vi "Point Data Updated.vi"(8 "error in":errorcluster, 9 "Data":variant, 10 "Point Ident":string, 11 "Sample Photosensor PID Flowsensor PID in":refnum<class "Sample Photosensor PID Flowsensor PID.lvclass">) -> (0 "error out":errorcluster, 3 "Sample Photosensor PID Flowsensor PID out":refnum<class "Sample Photosensor PID Flowsensor PID.lvclass">)   [LabVIEW 2023, in "Sample Photosensor PID Flowsensor PID.lvlib" / "Sample Photosensor PID Flowsensor PID.lvclass"]
uses:
  Sample Photosensor PID Flowsensor PID.lvclass
  Sample Photosensor PID Flowsensor PID.lvclass/Sample Photosensor PID Flowsensor PID.ctl
  <vilib>/Utility/error.llb/Error Cluster From Error Code.vi
  <vilib>/ErrorRing/Error Ring.xnode
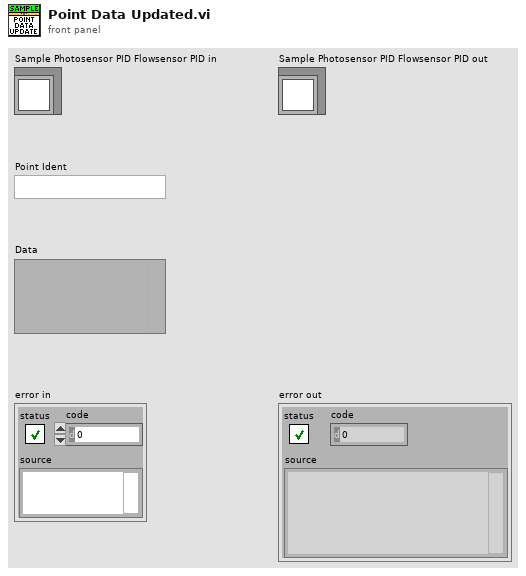
[diagram p1: front panel]
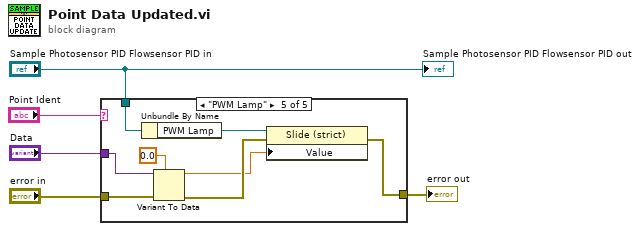
[diagram p0: block diagram]
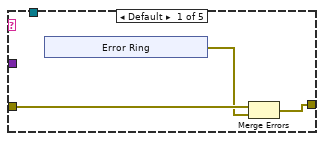
[diagram p2: hidden frame]
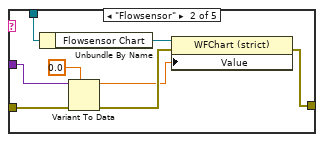
[diagram p3: hidden frame]
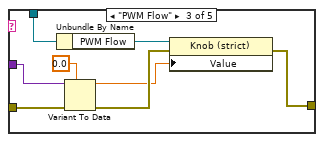
[diagram p4: hidden frame]
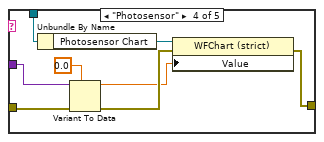
[diagram p5: hidden frame]
diagram:
  n1 = case shown="\"PWM Lamp\"" "Point Ident" {
    tunnel: "Data" -> [_ w16 w24 w32 w41]
    tunnel: "Sample Photosensor PID Flowsensor PID in" -> [_ w21 w29 w34 w40]
    tunnel: "error in" -> [w8 w19 w27 w33 w42]
    tunnel: [w6 w18 w22 w30 w38] -> w1
    frame Default {
      n2 = xnode "Error Ring"() -> ("error out"=w7:errorcluster)
      n3 = Merge Errors(w8, w7) -> (w6:errorcluster)
    }
    frame "Flowsensor" {
      n4 = Unbundle By Name(w21) -> ("Flowsensor Chart"=w20:refnum<vi>)
      n5 = Variant To Data(error in=w19, type=0.0, Variant=w16) -> (data=w14:dbl, error out=w17:errorcluster)
      n6 = property class="WFChart (strict)"(reference=w20, error in=w17, "Value"=w14) -> (error out=w18:errorcluster)  [unwired: 1 out]
    }
    frame "PWM Flow" {
      n7 = Unbundle By Name(w29) -> ("PWM Flow"=w28:refnum<vi>)
      n8 = Variant To Data(error in=w27, type=0.0, Variant=w24) -> (data=w23:dbl, error out=w26:errorcluster)
      n9 = property class="Knob (strict)"(reference=w28, error in=w26, "Value"=w23) -> (error out=w22:errorcluster)  [unwired: 1 out]
    }
    frame "Photosensor" {
      n10 = Unbundle By Name(w34) -> ("Photosensor Chart"=w37:refnum<vi>)
      n11 = Variant To Data(error in=w33, type=0.0, Variant=w32) -> (data=w35:dbl, error out=w36:errorcluster)
      n12 = property class="WFChart (strict)"(reference=w37, error in=w36, "Value"=w35) -> (error out=w30:errorcluster)  [unwired: 1 out]
    }
    frame "PWM Lamp" {
      n13 = Unbundle By Name(w40) -> ("PWM Lamp"=w45:refnum<vi>)
      n14 = Variant To Data(error in=w42, type=0.0, Variant=w41) -> (data=w43:dbl, error out=w44:errorcluster)
      n15 = property class="Slide (strict)"(reference=w45, error in=w44, "Value"=w43) -> (error out=w38:errorcluster)  [unwired: 1 out]
    }
  }
  "error out" <- w1
  "Sample Photosensor PID Flowsensor PID out" <- "Sample Photosensor PID Flowsensor PID in"
